vi "PH_BlackBox.set GUI element captions.vi"(0 "i ref in":refnum<vi>, 5 "error in (no error)":errorcluster) -> (14 "i ref out":refnum<vi>, 19 "error out":errorcluster)   [LabVIEW 2014, in "PH_BlackBox.lvlib"]
doc: "This VI sets GUI front panel element captions as it got it from data base."
uses:
  PH_BlackBox.lvlib
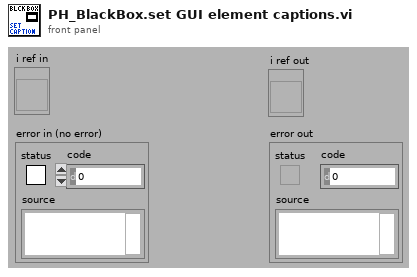
[diagram p1: front panel]
types:
  T1 = typedef "PH_BlackBox.lvlib/PH_BlackBox.i attribute.ctl" = cluster{"BB Remote Controlled?":bool, "GUI Refs":T2, "Position IN":T3, "Position OUT":T3, "BB Remote Controlled by other Instance?":bool, "Recipient":string, "Number":i32, "Caption Move":string, "Caption Out":string, "Caption In":string}
  T2 = typedef "PH_BlackBox.lvlib/PH_BlackBox.GUI Refs.ctl" = cluster{"MOVE IN":refnum<vi>, "MOVE":refnum<vi>, "IN":refnum<vi>, "OUT":refnum<vi>, "REMOTE":refnum<vi>, "GUI-Knob Move":refnum<vi>, "GUI-Knob Move in":refnum<vi>, "POWER ON":refnum<vi>, "Delete":refnum<vi>, "Function Textfield":refnum<vi>}
  T3 = typedef "PH_StatusHandler.lvlib/PH_StatusHandler.Status.ctl" = i16
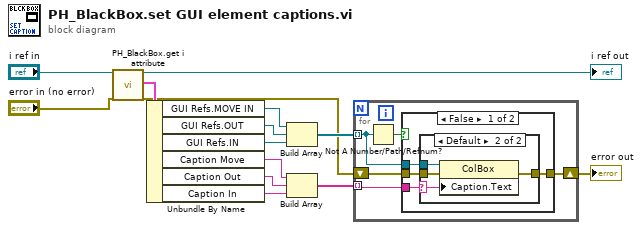
[diagram p0: block diagram]
diagram:
  n1 = call "PH_BlackBox.get i attribute.vi"("i ref in"="i ref in", "error in (no error)"="error in (no error)") -> ("i ref out"=→"i ref out":refnum<vi>, "i attribute"=w14:T1, "error out"=w1:errorcluster)  [unwired: 15 in]
  n2 = Unbundle By Name(w14) -> ("GUI Refs.MOVE IN"=w8:refnum<vi>, "GUI Refs.OUT"=w10:refnum<vi>, "GUI Refs.IN"=w9:refnum<vi>, "Caption Move"=w5:string, "Caption Out"=w4:string, "Caption In"=w3:string)
  n3 = Build Array(w8, w10, w9) -> (w7:refnum<vi>[])
  n4 = Build Array(w5, w4, w3) -> (w6:string[])
  n5 = for {
    tunnel: w7 -> [w16] mode=indexing
    tunnel: w6 -> [w15] mode=indexing
    shift-right: [w17] -> w11
    shift-left: w1 -> [w18]
    n6 = Not A Number/Path/Refnum?(number/path/refnum=w16) -> (NaN/Path/Refnum?=w19:bool)
    n7 = case shown="False" w19 {
      tunnel: w15 -> [w20 _]
      tunnel: [w23 w29] -> w17
      tunnel: w18 -> [w22 w29]
      tunnel: w16 -> [w21 _]
      frame False {
        n8 = case shown="Default" w20 {
          selector: w20 -> [_ w25]
          tunnel: w21 -> [_ w28]
          tunnel: w22 -> [w24 w27]
          tunnel: [w24 w26] -> w23
          frame "", "N/A" {
          }
          frame Default {
            n9 = property class="ColBox"(reference=w28, error in=w27, "Caption.Text"=w25) -> (error out=w26:errorcluster)  [unwired: 1 out]
          }
        }
      }
      frame True {
      }
    }
  }
  "error out" <- w11
